vi "Set Exclusions.vi"(4 "Exclude dependent shared libraries":bool, 6 "Exclude dependent packed libraries":bool, 8 "error in (no error)":errorcluster, 9 "Disconnect inline subVIs (F)":bool, 10 "Exclusions":T1={"Disconnect type definitions"=FALSE, "Remove unused polymorphic VI instances"=TRUE, "Remove unused members of project libraries"=TRUE, "Modify project library file after removing unused members"=TRUE}, 11 "PPL in":refnum<class "NI_AB_API_DPPL.lvclass">) -> (0 "error out":errorcluster, 3 "PPL out":refnum<class "NI_AB_API_DPPL.lvclass">)   [LabVIEW 2020, in "NI_AB_API_DPPL.lvclass"]
uses:
  <vilib>/AppBuilder/AB_API/DPPL/NI_AB_API_DPPL.lvclass
  <vilib>/AppBuilder/AB_API/common/AB_API Primary Exclusions.ctl
  <vilib>/AppBuilder/AB_API/PPL/NI_AB_API_PPL.lvclass
panel:
  # "^ unsupported for packed project libraries"
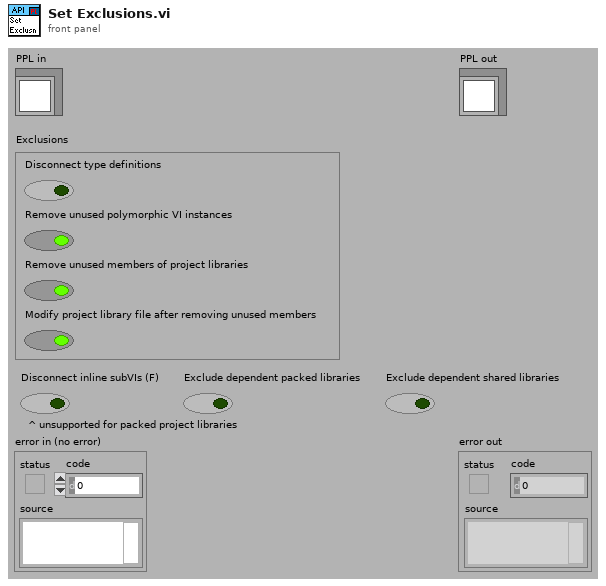
[diagram p1: front panel]
types:
  T1 = typedef "AB_API Primary Exclusions.ctl" = cluster{"Disconnect type definitions":bool, "Remove unused polymorphic VI instances":bool, "Remove unused members of project libraries":bool, "Modify project library file after removing unused members":bool}
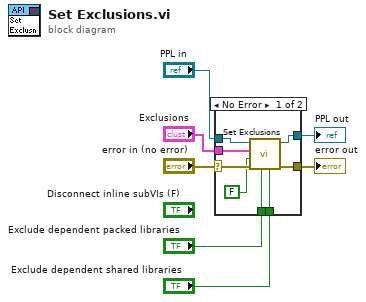
[diagram p0: block diagram]
diagram:
  n1 = case shown="No Error" "error in (no error)" {
    selector: "error in (no error)" -> [w13 w17]
    tunnel: [w12 w17] -> w6
    tunnel: [w14 w16] -> w4
    tunnel: "PPL in" -> [w15 w16]
    tunnel: "Exclusions" -> [w11 _]
    tunnel: "Exclude dependent packed libraries" -> [w9 _]
    tunnel: "Exclude dependent shared libraries" -> [w8 _]
    frame No Error {
      n2 = call-parent "Set Exclusions.vi"("Exclude dependent shared libraries"=w8, "Exclude dependent packed libraries"=w9, "error in (no error)"=w13, "Disconnect inline subVIs (F)"=FALSE, "Exclusions"=w11, "PPL in"=w15) -> ("error out"=w12:errorcluster, "PPL out"=w14:refnum<class "NI_AB_API_DPPL.lvclass">)  [unwired: 4 in]
    }
    frame Error {
    }
  }
  "error out" <- w6
  "PPL out" <- w4
